vi "Phasor Explorer.vi"() -> ()   [LabVIEW 2019]
uses:
  Decay & Gates Options.ctl
  SEPXP Phasor Plot Info.ctl
  Pseudo Phasor Parameters.ctl
  Phasor Explorer Display Parameters.ctl
  Type of Series.ctl
  Phasor Explorer Phasor Parameters.ctl
  Phasor Calculation Type.ctl
  Phasor Type.ctl
  Phasor Explorer Decay Parameters.ctl
  IRF Model.ctl
  Phasor Explorer Gate Parameters.ctl
  Gate Type.ctl
  Phasor Explorer Detector Parameters.ctl
  SEPXP Q [Element].ctl
  SEPXP Q [Event] List.ctl
  PhXP Internal Variables.ctl
  XY Plot Data.ctl
  XY Graph Plot Properties.ctl
  Cursor Info.ctl
  <vilib>/Utility/miscctls.llb/LVPointDoubleTypeDef.ctl
  SEPXP Globals.vi
  Notebook Main VI Name.vi
  User-defined Gate.vi
  Plot Editor.lvlib
  Notebook.lvlib
  XY Graph Add-Ons.lvlib
  Rich Text Box.lvlib
  Variant to Data.lvlib
panel:
  in  "Abort":bool
  in  "Message":string
  in  "Animated Busy Icon":bool=TRUE
  in  "Display Tabs":T1(tab)
  in  "Show UC Ticks":bool
  out "original tau_m":dbl[unit] format="%#_5g"
  out "original  tau_ph":dbl[unit] format="%#_5g"
  out "Phasor Graph TipStrip":string
  out "current tau_m":dbl[unit] format="%#_5g"
  out "current tau_ph":dbl[unit] format="%#_5g"
  out "tau_i":dbl[unit] format="%#_5g"
  out "Phasor Graph":cluster{"X Array":dbl[], "Y Array":dbl[]}[](graph)
  out "f(tau) Graph TipStrip":string
  out "Numerical Solution":T2 {"Solution 2" format="%#_5g"; "Solution 1" format="%#_5g"}
  out "Analytical Solutions":T2 caption="Analytical Solution" {"Solution 2" format="%#_5g"; "Solution 1" format="%#_5g"}
  in  "Use Cursor":bool caption="Use Pseudo Phasor Graph Cursor"
  in  "Linear Coefficients":cluster{"u":dbl, "v":dbl} {"v" format="%#_5g"; "u" format="%#_5g"}
  out "f(tau) Graph":cluster{"X Array":dbl[], "Y Array":dbl[]}[](graph)
  out "a(b) Graph TipStrip":string
  out "Max Tau":dbl[unit] format="%#_5g"
  out "Min Tau":dbl[unit] format="%#_5g"
  out "a(b) Graph":cluster{"X Array":dbl[], "Y Array":dbl[]}[](graph)=[{"X Array"=[0.0, 0.01, 0.02, 0.03, 0.04, 0.05, 0.060000000000000005, 0.07, 0.08, 0.09, 0.09999999999999999, 0.10999999999999999, 0.11999999999999998, 0.12999999999999998, 0.13999999999999999, 0.15, 0.16, 0.17, 0.18000000000000002, 0.19000000000000003, 0.20000000000000004, 0.21000000000000005, 0.22000000000000006, 0.23000000000000007, 0.24000000000000007, 0.25000000000000006, 0.26000000000000006, 0.2700000000000001, 0.2800000000000001, 0.2900000000000001, 0.3000000000000001, 0.3100000000000001, 0.3200000000000001, 0.3300000000000001, 0.34000000000000014, 0.35000000000000014, 0.36000000000000015, 0.37000000000000016, 0.38000000000000017, 0.3900000000000002, 0.4000000000000002, 0.4100000000000002, 0.4200000000000002, 0.4300000000000002, 0.4400000000000002, 0.45000000000000023, 0.46000000000000024, 0.47000000000000025, 0.48000000000000026, 0.49000000000000027, 0.5000000000000002, 0.5100000000000002, 0.5200000000000002, 0.5300000000000002, 0.5400000000000003, 0.5500000000000003, 0.5600000000000003, 0.5700000000000003, 0.5800000000000003, 0.5900000000000003, 0.6000000000000003, 0.6100000000000003, 0.6200000000000003, 0.6300000000000003, 0.6400000000000003, 0.6500000000000004, 0.6600000000000004, 0.6700000000000004, 0.6800000000000004, 0.6900000000000004, 0.7000000000000004, 0.7100000000000004, 0.7200000000000004, 0.7300000000000004, 0.7400000000000004, 0.7500000000000004, 0.7600000000000005, 0.7700000000000005, 0.7800000000000005, 0.7900000000000005, 0.8000000000000005, 0.8100000000000005, 0.8200000000000005, 0.8300000000000005, 0.8400000000000005, 0.8500000000000005, 0.8600000000000005, 0.8700000000000006, 0.8800000000000006, 0.8900000000000006, 0.9000000000000006, 0.9100000000000006, 0.9200000000000006, 0.9300000000000006, 0.9400000000000006, 0.9500000000000006, 0.9600000000000006, 0.9700000000000006, 0.9800000000000006, 0.9900000000000007, 1.0000000000000007], "Y Array"=[0.0, 0.01, 0.02, 0.03, 0.04, 0.05, 0.060000000000000005, 0.07, 0.08, 0.09, 0.09999999999999999, 0.10999999999999999, 0.11999999999999998, 0.12999999999999998, 0.13999999999999999, 0.15, 0.16, 0.17, 0.18000000000000002, 0.19000000000000003, 0.20000000000000004, 0.21000000000000005, 0.22000000000000006, 0.23000000000000007, 0.24000000000000007, 0.25000000000000006, 0.26000000000000006, 0.2700000000000001, 0.2800000000000001, 0.2900000000000001, 0.3000000000000001, 0.3100000000000001, 0.3200000000000001, 0.3300000000000001, 0.34000000000000014, 0.35000000000000014, 0.36000000000000015, 0.37000000000000016, 0.38000000000000017, 0.3900000000000002, 0.4000000000000002, 0.4100000000000002, 0.4200000000000002, 0.4300000000000002, 0.4400000000000002, 0.45000000000000023, 0.46000000000000024, 0.47000000000000025, 0.48000000000000026, 0.49000000000000027, 0.5000000000000002, 0.5100000000000002, 0.5200000000000002, 0.5300000000000002, 0.5400000000000003, 0.5500000000000003, 0.5600000000000003, 0.5700000000000003, 0.5800000000000003, 0.5900000000000003, 0.6000000000000003, 0.6100000000000003, 0.6200000000000003, 0.6300000000000003, 0.6400000000000003, 0.6500000000000004, 0.6600000000000004, 0.6700000000000004, 0.6800000000000004, 0.6900000000000004, 0.7000000000000004, 0.7100000000000004, 0.7200000000000004, 0.7300000000000004, 0.7400000000000004, 0.7500000000000004, 0.7600000000000005, 0.7700000000000005, 0.7800000000000005, 0.7900000000000005, 0.8000000000000005, 0.8100000000000005, 0.8200000000000005, 0.8300000000000005, 0.8400000000000005, 0.8500000000000005, 0.8600000000000005, 0.8700000000000006, 0.8800000000000006, 0.8900000000000006, 0.9000000000000006, 0.9100000000000006, 0.9200000000000006, 0.9300000000000006, 0.9400000000000006, 0.9500000000000006, 0.9600000000000006, 0.9700000000000006, 0.9800000000000006, 0.9900000000000007, 1.0000000000000007]}]
  in  "Compute Delta Tau":bool
  out "Pseudo-Phase Lifetime Graph TipStrip":string
  out "Pseudo-Phase Lifetime Graph":cluster{"X Array":dbl[], "Y Array":dbl[]}[](graph)=[{"X Array"=[0.0, 1.0, 2.0, 3.0, 4.0, 5.0, 6.0, 7.0, 8.0, 9.0, 10.0, 11.0, 12.0, 13.0, 14.0, 15.0, 16.0, 17.0, 18.0, 19.0, 20.0, 21.0, 22.0, 23.0, 24.0, 25.0, 26.0, 27.0, 28.0, 29.0, 30.0, 31.0, 32.0, 33.0, 34.0, 35.0, 36.0, 37.0, 38.0, 39.0, 40.0, 41.0, 42.0, 43.0, 44.0, 45.0, 46.0, 47.0, 48.0, 49.0, 50.0, 51.0, 52.0, 53.0, 54.0, 55.0, 56.0, 57.0, 58.0, 59.0, 60.0, 61.0, 62.0, 63.0, 64.0, 65.0, 66.0, 67.0, 68.0, 69.0, 70.0, 71.0, 72.0, 73.0, 74.0, 75.0, 76.0, 77.0, 78.0, 79.0, 80.0, 81.0, 82.0, 83.0, 84.0, 85.0, 86.0, 87.0, 88.0, 89.0, 90.0, 91.0, 92.0, 93.0, 94.0, 95.0, 96.0, 97.0, 98.0, 99.0, 100.0], "Y Array"=[0.0, 1.0, 2.0, 3.0, 4.0, 5.0, 6.0, 7.0, 8.0, 9.0, 10.0, 11.0, 12.0, 13.0, 14.0, 15.0, 16.0, 17.0, 18.0, 19.0, 20.0, 21.0, 22.0, 23.0, 24.0, 25.0, 26.0, 27.0, 28.0, 29.0, 30.0, 31.0, 32.0, 33.0, 34.0, 35.0, 36.0, 37.0, 38.0, 39.0, 40.0, 41.0, 42.0, 43.0, 44.0, 45.0, 46.0, 47.0, 48.0, 49.0, 50.0, 51.0, 52.0, 53.0, 54.0, 55.0, 56.0, 57.0, 58.0, 59.0, 60.0, 61.0, 62.0, 63.0, 64.0, 65.0, 66.0, 67.0, 68.0, 69.0, 70.0, 71.0, 72.0, 73.0, 74.0, 75.0, 76.0, 77.0, 78.0, 79.0, 80.0, 81.0, 82.0, 83.0, 84.0, 85.0, 86.0, 87.0, 88.0, 89.0, 90.0, 91.0, 92.0, 93.0, 94.0, 95.0, 96.0, 97.0, 98.0, 99.0, 100.0]}]
  out "Decay & Gates Graph TipStrip":string
  in  "Decay & Gates Options":T3
  out "Decay & Gates Graph":cluster{"X Array":dbl[], "Y Array":dbl[]}[](graph)
  in  "Version":enum32{"Version 1", "Version 2"}(radio)=enum."Version 2"
  out "Sum of Gates Graph TipStrip":string
  out "Sum of Gates Graph":cluster{"X Array":dbl[], "Y Array":dbl[]}[](graph)
  out "Phasor Graph Plots Metadata":T4[](array[typedef]) {"Phasor Explorer Parameters"."Detector Parameters"."Frames/Image" min=1; "Phasor Explorer Parameters"."Detector Parameters"."Multiplicity" min=0; "Phasor Explorer Parameters"."Detector Parameters"."Bits/Frame" min=1; "Phasor Explorer Parameters"."Detector Parameters"."Gates/Frame" min=1; "Phasor Explorer Parameters"."Gate Parameters"."# Steps" min=0.0; "Phasor Explorer Parameters"."Gate Parameters"."Tolerance" min=0.0; "Phasor Explorer Parameters"."Gate Parameters"."Top Slope" min=0.0; "Phasor Explorer Parameters"."Gate Parameters"."Edge Width" min=0.0; "Phasor Explorer Parameters"."Gate Parameters"."Gate Step" min=0.0; "Phasor Explorer Parameters"."Gate Parameters"."# Gates" min=0.0 step=1.0; "Phasor Explorer Parameters"."Gate Parameters"."Gate Width" min=0.0; "Phasor Explorer Parameters"."Decay & IRF Parameters"."Lifetime" min=0.0; "Phasor Explorer Parameters"."Decay & IRF Parameters"."Laser Period" min=0.0; "Phasor Explorer Parameters"."Phasor Parameters"."Square Gate Width" min=0.0; "Phasor Explorer Parameters"."Phasor Parameters"."# Gates" min=0.0; "Phasor Explorer Parameters"."Phasor Parameters"."Calibration Lifetime" min=0.0; "Phasor Explorer Parameters"."Phasor Parameters"."Harmonic frequency" min=0.0; "Phasor Explorer Parameters"."Display Parameters"."Min tau" min=0.0; "Phasor Explorer Parameters"."Display Parameters"."Max tau" min=0.0; "Phasor Explorer Parameters"."Display Parameters"."# Points" min=1 step=1}
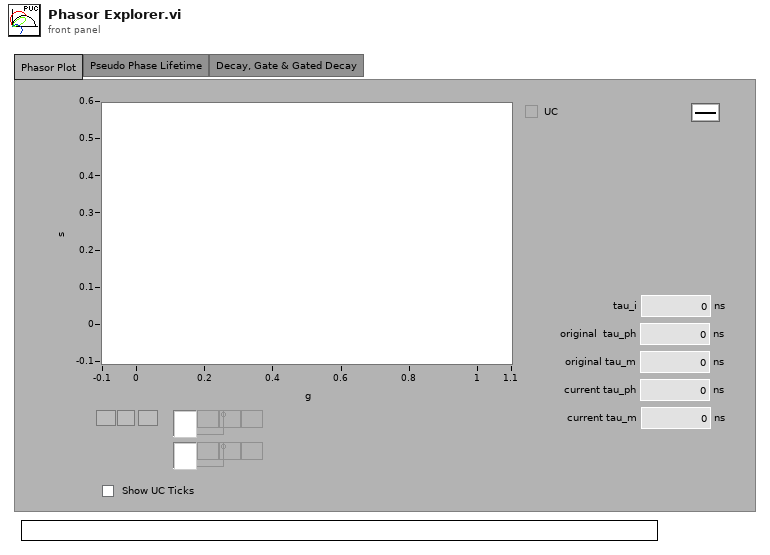
[diagram p1: front panel]
types:
  T1 = enum32{"Phasor Plot", "UC Intersections", "Alpha vs Beta", "Pseudo Phase Lifetime", "Decay, Gate & Gated Decay", "Sum of Gates", "Debug"}
  T2 = cluster{"Solution 1":dbl[unit], "Solution 2":dbl[unit]}
  T3 = typedef "Decay & Gates Options.ctl" = cluster{"Decay":bool, "Gate":bool, "Gated Decay":bool}
  T4 = typedef "SEPXP Phasor Plot Info.ctl" = cluster{"Lifetime/Fraction Array":dbl[], "Phasor Explorer Parameters":T5, "Phase Lifetimes":dbl[], "Modulus Lifetimes":dbl[]}
  T5 = typedef "Pseudo Phasor Parameters.ctl" = cluster{"Display Parameters":T6, "Phasor Parameters":T8, "Decay & IRF Parameters":T11, "Gate Parameters":T13, "Detector Parameters":T15}
  T6 = typedef "Phasor Explorer Display Parameters.ctl" = cluster{"# Points":i32, "Ramp Type":enum16{"Linear", "Logarithmic"}, "Type of Series":T7, "Min tau":dbl[unit], "Max tau":dbl[unit], "Include 0":bool, "Include Infinity":bool}
  T7 = typedef "Type of Series.ctl" = enum16{"1-Exp Decays", "Linear Combination of 1-Exp"}
  T8 = typedef "Phasor Explorer Phasor Parameters.ctl" = cluster{"Harmonic frequency":dbl[unit], "Use f* = 1/D Frequency":bool, "Calibrated Phasor":bool, "Calibration Lifetime":dbl[unit], "Phasor Calculation":T9, "SEPL Type":T10, "# Gates":dbl, "Square Gate Width":dbl[unit], "Show Ticks":bool}
  T9 = typedef "Phasor Calculation Type.ctl" = enum16{"Direct Sum", "Analytical Formula"}
  T10 = typedef "Phasor Type.ctl" = enum16{"UC", "L_N", "L_N[W]"}
  T11 = typedef "Phasor Explorer Decay Parameters.ctl" = cluster{"Lifetime":dbl[unit], "IRF Offset":dbl[unit], "Laser Period":dbl[unit], "Normalized Decays":bool, "IRF Model":T12, "IRF Parameter 1":dbl[unit]}
  T12 = typedef "IRF Model.ctl" = enum16{"Dirac", "Exponential"}
  T13 = typedef "Phasor Explorer Gate Parameters.ctl" = cluster{"First Gate Start":dbl[unit], "Use Gate Center":bool, "Gate Width":dbl[unit], "Gate Step":dbl[unit], "# Gates":dbl, "Gate Type":T14, "Edge Width":dbl[unit], "Top Slope":dbl[unit], "Reversed Sawtooth?":bool, "Analytical Computation":bool, "Tolerance":dbl, "Integration":enum32{"Item 0", "Item 1"}, "# Steps":dbl, "Type of User-defined Function":enum32{"Gate", "IRF"}}
  T14 = typedef "Gate Type.ctl" = enum16{"Square", "Finite Edge Square", "Finite Edge, Tilted Top Square", "Triangle", "Sawtooth", "User-defined"}
  T15 = typedef "Phasor Explorer Detector Parameters.ctl" = cluster{"Frames/Image":i32, "Gates/Frame":i32, "Bits/Frame":i32, "Multiplicity":i32, "Incident Signal":dbl}
  T16 = enum32{"Phasor Plot", "UC Intersections", "Alpha vs Beta", "Pseudo Phase Lifetime", "Decay, Gate & Gated Decay", "Sum of Gates", "Debug"}[]
  T17 = typedef "PhXP Internal Variables.ctl" = cluster{"User-Defined Gate":T18, "User-defined Gate Plot Style":T19}
  T18 = typedef "XY Plot Data.ctl" = cluster{"X Array":dbl[], "Y Array":dbl[]}
  T19 = typedef "XY Graph Plot Properties.ctl" = cluster{"Plot Index":i32, "Plot.Bar Plot Style":u8, "Plot.DigitalLineStyle":u8, "Plot.TransitionLocation":u8, "Plot.Transition Type":u8, "Plot.Fill To":i16, "Plot.Fill/Pt. Color":u32, "Plot.Label Format":u8, "Plot.Line Style":u8, "Plot.Line Width":u8, "Plot.Plot Color":u32, "Plot.Plot Interpolation":u8, "Plot.Plot Name":string, "Plot.Point Style":u8, "Plot.Visible?":bool, "Plot.XScaleIdx":u32, "Plot.YScaleIdx":u32, "Plot.Anti-aliased":bool}
  T20 = typedef "SEPXP Q [Element].ctl" = cluster{"SEPXP Q Event":T21, "Data":variant}
  T21 = typedef "SEPXP Q [Event] List.ctl" = enum16{"Idle", "Initialization", "Show-Hide UC Ticks", "Edit User-defined Gate", "Update Phasor Graph", "Update Sum of Gates Graph", "Update Parameters", "Compute Decay &/or Gates", "Find Pseudo UC Intersections", "Compute alpha(beta) Plot", "Compute Pseudo-Phase Lifetime Plot", "Export Parameters to Clipboard", "Update Phase & Modulus Lifetime", "XY Graph Special Event", "Update Graph Plots Info", "Fit to Circle", "Quit"}
  T22 = typedef "SEPXP Tipstrip Event Registration Refnums.ctl" = cluster{"Phasor Graph Event Registration Refnum":refnum<event-registration>, "Sum of Gates Graph Event Registration Refnum":refnum<event-registration>, "f(tau) Graph Event Registration Refnum":refnum<event-registration>, "a(b) Graph Event Registration Refnum":refnum<event-registration>, "Pseudo-Phase Lifetime Graph Event Registration Refnum":refnum<event-registration>, "Decay & Gate Graph Event Registration Refnum":refnum<event-registration>}
  T23 = enum32{"Phasor Plot", "UC Intersections", "Alpha vs Beta", "Pseudo Phase Lifetime", "Decay, Gate & Gated Decay", "Sum of Gates"}
  T24 = typedef "Cursor Info.ctl" = cluster{"CtlRef":refnum<vi>, "CursIdx":i32, "CursRef":refnum<vi>, "PlotIdx":i32, "PointIdx":i32, "CursLoc":cluster{"X":dbl, "Y":dbl}}
  T25 = typedef "XY Graph Event.ctl" = cluster{"ItemTag":string, "CtlRef":refnum<vi>, "Coords":T26}
  T26 = typedef "LVPoint32TypeDef.ctl" = cluster{"Horizontal":i32, "Vertical":i32}
  T27 = typedef "LVPointDoubleTypeDef.ctl" = cluster{"X":dbl, "Y":dbl}
  T28 = cluster{"XY Graph Ref":refnum<vi>, "Mouse Coordinates":T27, "Plot Index":i32}
  T29 = typedef "Rich Text Box.lvlib/Text Formatting.ctl" = cluster{"Font":string, "Text Color":T30, "Text Background Color":T30, "Text Style":enum16{"Regular", "Bold", "Italic", "Underline", "Strikeout"}, "Font Size (Points)":dbl, "Text Alignment":i32}
  T30 = typedef "Rich Text Box.lvlib/Text Colors.ctl" = enum16{"Unchanged", "Black", "Blue", "Gray", "Green", "Red", "White"}
  T31 = cluster{"ItemTag":string, "CtlRef":refnum<vi>, "Coords":T26}
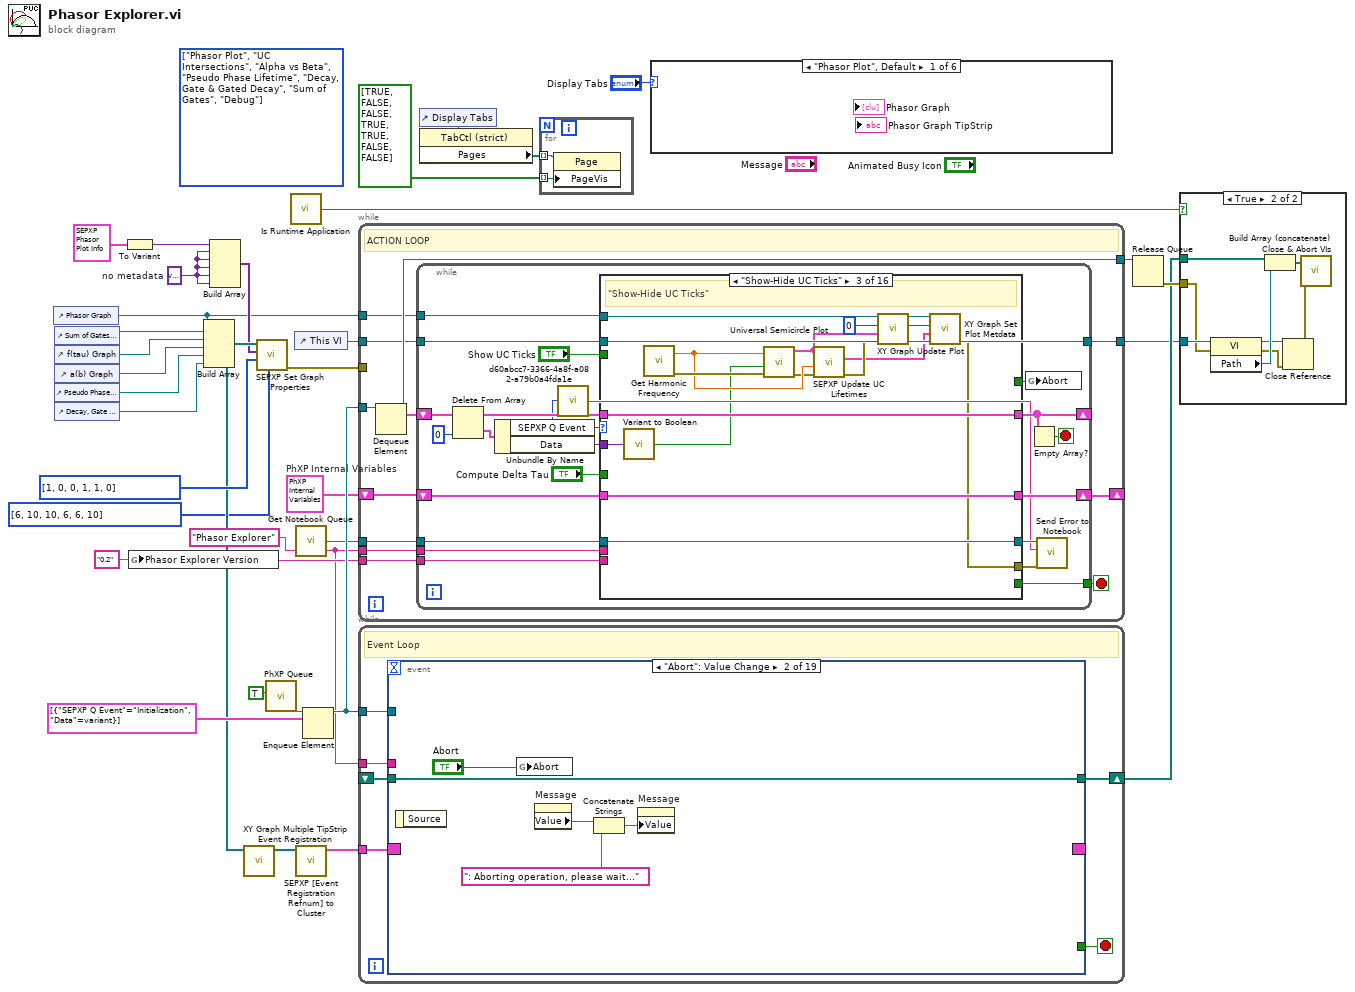
[diagram p0: block diagram]
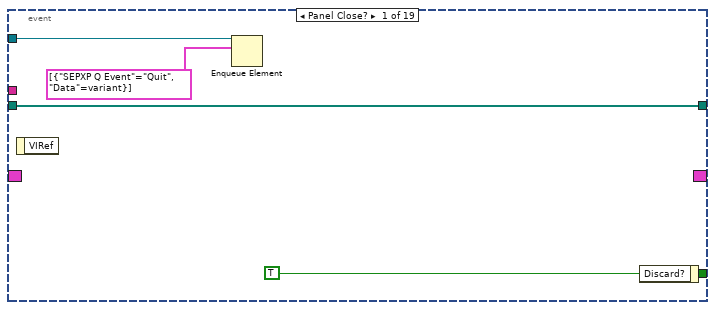
[diagram p3: hidden frame]
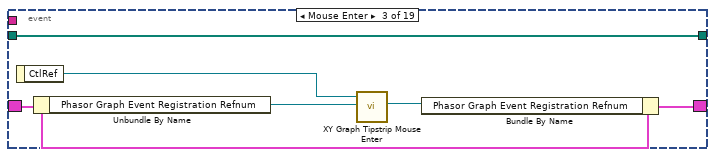
[diagram p4: hidden frame]
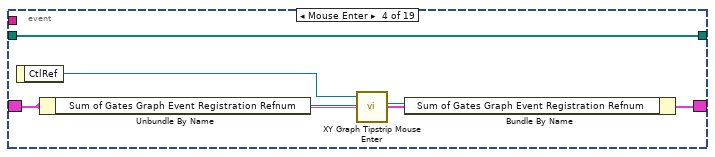
[diagram p5: hidden frame]
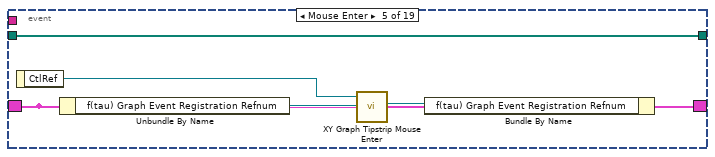
[diagram p6: hidden frame]
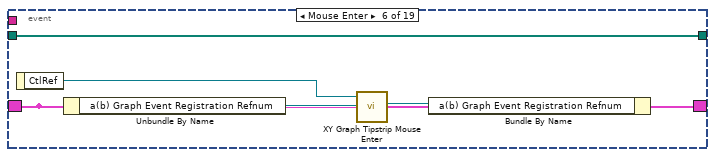
[diagram p7: hidden frame]
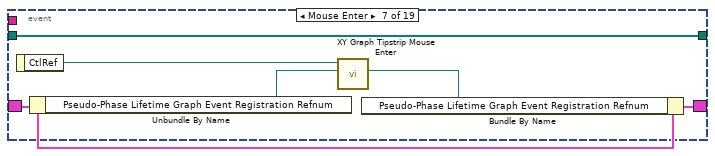
[diagram p8: hidden frame]
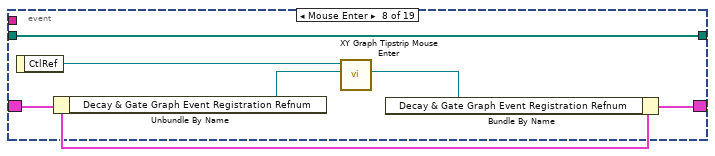
[diagram p9: hidden frame]
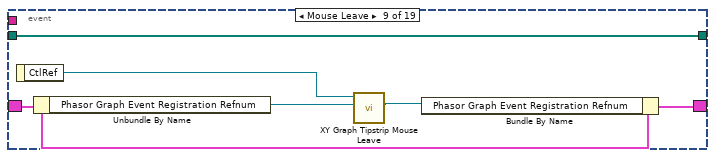
[diagram p10: hidden frame]
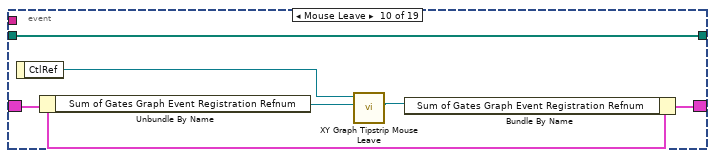
[diagram p11: hidden frame]
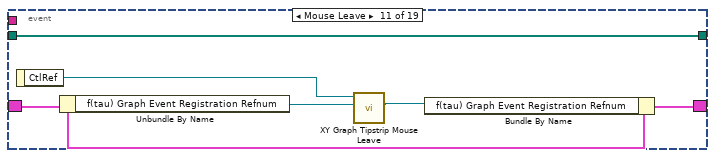
[diagram p12: hidden frame]
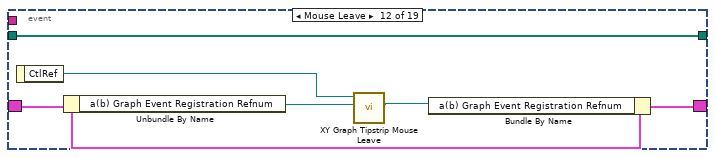
[diagram p13: hidden frame]
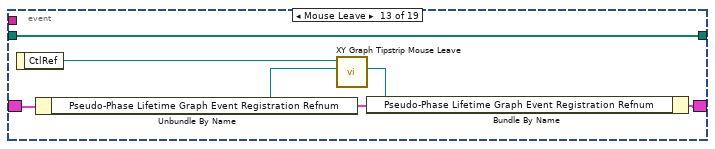
[diagram p14: hidden frame]
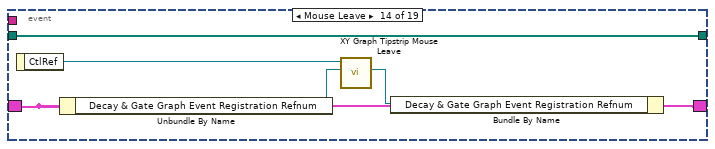
[diagram p15: hidden frame]
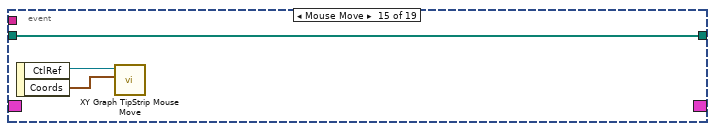
[diagram p16: hidden frame]
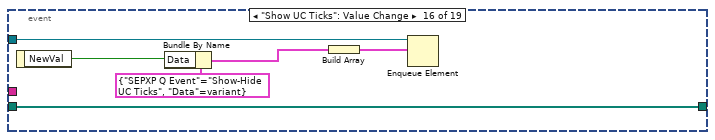
[diagram p17: hidden frame]
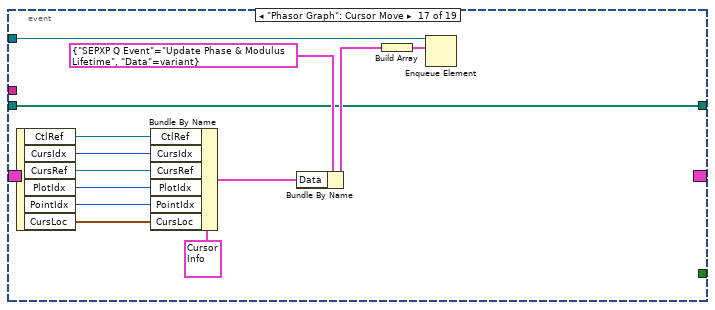
[diagram p18: hidden frame]
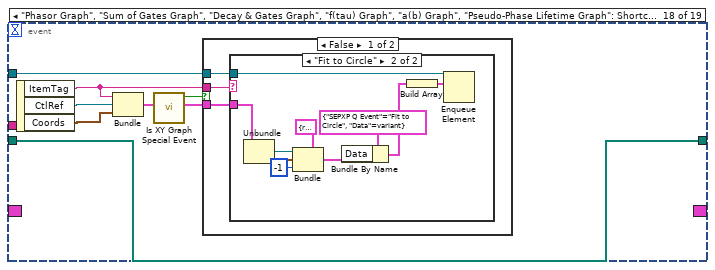
[diagram p19: hidden frame]
diagram:
  (unwired) T16 [enum."Phasor Plot", enum."UC Intersections", enum."Alpha vs Beta", enum."Pseudo Phase Lifetime", enum."Decay, Gate & Gated Decay", enum."Sum of Gates", enum."Debug"] items=["Phasor Plot", "UC Intersections", "Alpha vs Beta", "Pseudo Phase Lifetime", "Decay, Gate & Gated Decay", "Sum of Gates", "Debug"] ("Display Tabs")
  w9 = variant  # no metadata
  w15 = "Phasor Explorer" ("Phasor Explorer Version")
  w28 = "0.2" ("Phasor Explorer Version")
  w31 = T17 {"User-Defined Gate"={"X Array"=[], "Y Array"=[]}, "User-defined Gate Plot Style"={"Plot Index"=0, "Plot.Bar Plot Style"=0, "Plot.DigitalLineStyle"=0, "Plot.TransitionLocation"=0, "Plot.Transition Type"=0, "Plot.Fill To"=-1, "Plot.Fill/Pt. Color"=0, "Plot.Label Format"=0, "Plot.Line Style"=0, "Plot.Line Width"=0, "Plot.Plot Color"=0, "Plot.Plot Interpolation"=4, "Plot.Plot Name"="User-defined Gate", "Plot.Point Style"=0, "Plot.Visible?"=TRUE, "Plot.XScaleIdx"=0, "Plot.YScaleIdx"=0, "Plot.Anti-aliased"=TRUE}}  # PhXP Internal Variables
  n1 = control-ref of="Phasor Graph"() -> (w8:refnum<vi>)
  n2 = control-ref of="Sum of Gates Graph"() -> (w26:refnum<vi>)
  n3 = control-ref of="f(tau) Graph"() -> (w25:refnum<vi>)
  n4 = control-ref of="a(b) Graph"() -> (w24:refnum<vi>)
  n5 = control-ref of="Pseudo Phase Lifetime Graph"() -> (w23:refnum<vi>)
  n6 = control-ref of="Decay, Gate & Gated Decay Graph"() -> (w22:refnum<vi>)
  n7 = To Variant(anything=T4 {"Lifetime/Fraction Array"=[], "Phasor Explorer Parameters"={"Display Parameters"={"# Points"=0, "Ramp Type"=enum."Linear", "Type of Series"=enum."1-Exp Decays", "Min tau"=0.0, "Max tau"=0.0, "Include 0"=FALSE, "Include Infinity"=FALSE}, "Phasor Parameters"={"Harmonic frequency"=0.0, "Use f* = 1/D Frequency"=FALSE, "Calibrated Phasor"=FALSE, "Calibration Lifetime"=1e-09, "Phasor Calculation"=enum."Direct Sum", "SEPL Type"=enum."UC", "# Gates"=1.0, "Square Gate Width"=1e-09, "Show Ticks"=FALSE}, "Decay & IRF Parameters"={"Lifetime"=0.0, "IRF Offset"=0.0, "Laser Period"=0.0, "Normalized Decays"=FALSE, "IRF Model"=enum."Dirac", "IRF Parameter 1"=0.0}, "Gate Parameters"={"First Gate Start"=0.0, "Use Gate Center"=FALSE, "Gate Width"=0.0, "Gate Step"=0.0, "# Gates"=0.0, "Gate Type"=enum."Square", "Edge Width"=0.0, "Top Slope"=0.0, "Reversed Sawtooth?"=FALSE, "Analytical Computation"=FALSE, "Tolerance"=1.0, "Integration"=enum."Item 0", "# Steps"=1.0, "Type of User-defined Function"=enum."Gate"}, "Detector Parameters"={"Frames/Image"=0, "Gates/Frame"=0, "Bits/Frame"=0, "Multiplicity"=0, "Incident Signal"=0.0}}, "Phase Lifetimes"=[], "Modulus Lifetimes"=[]} ("Phasor Graph Plot Info")) -> (Variant=w11:variant)
  n8 = global write "SEPXP Globals.vi" "Phasor Explorer Version"(w28) -> ()
  n9 = Build Array(w8, w26, w25, w24, w23, w22) -> (w19:refnum<vi>[])
  n10 = Build Array(w11, w9, w9, w9, w9, w9) -> (w10:variant[])
  n11 = call "XY Graph Multiple TipStrip Event Registration.vi"("XY Graph Refnums"=w19) -> ("Tipstrips Event Registrations"=w18:refnum<event-registration>[])  [unwired: 9 in, 1 out]
  n12 = call "SEPXP Set Graph Properties.vi"("Max Legend Size (8)"=i32[] [6, 10, 10, 6, 6, 10], "# Preserved PLots"=i32[] [1, 0, 0, 1, 1, 0], "Metadata Type"=w10, "XY Graph Ref Array"=w19) -> ("Error Out"=w21:errorcluster)  [unwired: 7 in]
  n13 = call "PhXP Queue.vi"("create if not found? (F)"=TRUE) -> ("PhXP Queue"=w14:refnum<queue>)  [unwired: 10 in]
  n14 = call "Is Runtime Application.vi"() -> ("Runtime ?"=w2:bool)  [unwired: 8 in, 1 out]
  n15 = control-ref of="This VI"() -> (w7:refnum<vi>)
  n16 = call "Get Notebook Queue.vi"() -> ("Notebook Queue"=w29:refnum<queue>)  [unwired: 9 in]
  n17 = call "SEPXP [Event Registration Refnum] to Cluster.vi"("Tipstrips Event Registrations"=w18) -> ("Tipstrip RE refnums"=w17:T22)  [unwired: 10 in]
  n18 = Enqueue Element(queue=w14, element=T20[] [{"SEPXP Q Event"=enum."Initialization", "Data"=variant}] ("PSEXP Q Element")) -> (queue out=w32:refnum<queue>)  [unwired: 2 in, 2 out]
  n19 = while {
    tunnel: w32 -> [w46]
    tunnel: [w44] -> w33
    tunnel: w7 -> [w42]
    shift-right: [w40] -> _
    shift-left: w31 -> [w41]
    tunnel: w29 -> [w39]
    tunnel: w28 -> [w38]
    tunnel: w15 -> [w37]
    tunnel: w21 -> [_]
    tunnel: w8 -> [w36]
    tunnel: [w35] -> w1
    stop <- w43 stop-if-true
    # "ACTION LOOP"
    n20 = Dequeue Element(queue=w46) -> (queue out=w44:refnum<queue>, element=w45:T20[])  [unwired: 2 in, 2 out]
    n21 = while {
      shift-right: [w64] -> _
      shift-left: w45 -> [w66]
      tunnel: [w62] -> w43
      tunnel: w42 -> [w47]
      shift-right: [w60] -> w40
      shift-left: w41 -> [w61]
      tunnel: w39 -> [w58]
      tunnel: w38 -> [w57]
      tunnel: w37 -> [w56]
      tunnel: w36 -> [w50]
      tunnel: [w47] -> w35
      stop <- w63 stop-if-true
      n22 = Delete From Array(array=w66, index=0) -> (deleted portion=w67:T20, array with subset deleted=w65:T20[])  [unwired: 1 in]
      n23 = Unbundle By Name(w67) -> ("SEPXP Q Event"=w52:T21, "Data"=w59:variant)
      n24 = call "d60abcc7-3366-4a8f-a082-a79b0a4fda1e.vi"("Enum"=w52) -> ("String"=w51:string)
      n25 = case shown="\"Show-Hide UC Ticks\"" w52 {
        tunnel: w65 -> [w71 w93 w121 w131 w144 w152 w164 w176 w185 w191 w201 w223 w232 w239 w250 _]
        tunnel: [w71 w93 w121 w131 w144 w152 w164 w176 w185 w191 w201 w223 w232 w239 w250 T20[] []] -> w64
        tunnel: [_ _ _ _ _ _ _ _ _ _ _ _ _ _ _ w252] -> w62
        tunnel: w47 -> [_ _ _ _ w141 w148 _ w167 w180 _ w195 w219 _ _ _ _]
        tunnel: w61 -> [w70 w77 w119 w128 w136 w149 w158 w173 w182 w188 w196 w220 w231 w238 w249 w258]
        tunnel: [w70 w77 w119 w129 w136 w149 w158 w173 w182 w188 w196 w220 w231 w238 w249 w258] -> w60
        tunnel: w59 -> [_ _ w108 _ _ _ w163 _ _ _ _ _ w228 _ w248 _]
        tunnel: w58 -> [w69 w84 w120 w122 w137 w145 w156 w165 w177 w186 w192 w202 w224 w237 w245 w254]
        tunnel: w57 -> [_ w92 _ _ _ _ _ _ _ _ _ _ _ _ _ w256]
        tunnel: w56 -> [_ w91 _ _ _ _ _ _ _ _ _ _ _ _ _ w257]
        tunnel: "Compute Delta Tau" -> [_ _ _ _ _ _ _ _ w179 _ _ _ _ _ _ _]
        tunnel: [_ w86 w112 w123 w138 w146 w157 w166 w178 w187 w193 w203 w225 _ w243 w251] -> w54
        tunnel: [w69 w84 w120 w122 w137 w145 w156 w165 w177 w186 w192 w202 w224 w237 w245 w254] -> w53
        tunnel: w50 -> [_ w82 w114 _ _ _ _ _ _ _ _ _ _ w236 _ _]
        tunnel: [_ _ _ _ FALSE ("Abort") _ _ _ _ _ _ _ _ _ _ _] -> w49
        tunnel: "Show UC Ticks" -> [_ w72 _ _ _ _ _ _ _ _ _ _ _ _ _ _]
        frame "Idle", Default {
          # "\"Idle\", Default"
        }
        frame "Initialization" {
          # "\"Initialization\""
          n26 = call "Send Start-Stop Message.vi"("Start(T)/Stop(F)"=TRUE, "Version number"=w92, "Software Name"=w91, "Notebook Queue"=w84) -> ("Error Out"=w85:errorcluster)  [unwired: 7 in]
          n27 = call "Save-Load PhXP Settings.vi"("Load(F)/Save (T)"=FALSE) -> ("Error Out"=w89:errorcluster)  [unwired: 9 in, 1 out]
          n28 = call "9d87ee79-5232-47ce-8c93-ac6730099a75.vi"("# Steps (1)"=100) -> ("Ramp"=w101:dbl[])  [unwired: 9 in, 1 out]
          n29 = call "79f5c63b-0c71-4b9b-95d4-cbcc2b15c9cb.vi"("# Steps (1)"=100, "End (1)"=100.0) -> ("Ramp"=w106:dbl[])  [unwired: 8 in, 1 out]
          n30 = call "Get Harmonic Frequency.vi"("Error In"=w89) -> ("Error Out"=w75:errorcluster, "Harmonic frequency"=w76:dbl[unit])  [unwired: 2 in, 1 out]
          n31 = Bundle("Ramp"=w101, "Ramp"=w101) -> (w103:cluster{"Ramp":dbl[], "Ramp":dbl[]})  [unwired: 1 in]
          n32 = Bundle("Ramp"=w106, "Ramp"=w106) -> (w104:cluster{"Ramp":dbl[], "Ramp":dbl[]})  [unwired: 1 in]
          n33 = call "Universal Semicircle Plot.vi"("Error In"=w75, "Show Ticks"=w72, "Harmonic frequency"=w76) -> ("Error Out"=w74:errorcluster, "Universal Semi-circle"=w80:cluster{"X Array":dbl[], "Y Array":dbl[]})  [unwired: 6 in, 1 out]
          n34 = Build Array(w103) -> (w102:cluster{"Ramp":dbl[], "Ramp":dbl[]}[])
          n35 = Build Array(w104) -> (w105:cluster{"Ramp":dbl[], "Ramp":dbl[]}[])
          n36 = call "SEPXP Update UC Lifetimes.vi"("Error In"=w74, "Harmonic Frequency"=w76, "Universal Semi-circle"=w80) -> ("Error Out"=w73:errorcluster, "PhXP UC Plot Info out"=w81:T4)  [unwired: 7 in]
          n37 = property on="a(b) Graph" class="XYGraph (strict)"("Value"=w102, "Active Plot"=u32 0, "Plot.Plot Name"="alpha = beta") -> ()  [unwired: 2 in, 2 out]
          n38 = property on="Pseudo-Phase Lifetime Graph" class="XYGraph (strict)"("Value"=w105, "Active Plot"=u32 0, "Plot.Plot Name"="tau = P-tau_ph") -> ()  [unwired: 2 in, 2 out]
          n39 = call "XY Graph Add Single Plot with Name.vi"("XYGraph Ref in"=w82, "Keep Existing Plots (T)"=FALSE, "Plot"=w80, "Plot Metadata"=w81, "Plot Name (\"Plot\")"="UC" ("Plot.Plot Name"), "error in (no error)"=w73) -> ("error out"=w78:errorcluster)  [unwired: 6 in, 3 out]
          n40 = Merge Errors(w78, w85) -> (w86:errorcluster)
          n41 = local write "Display Tabs"(T23."Phasor Plot" ("Display Tabs")) -> ()
        }
        frame "Show-Hide UC Ticks" {
          w111 = 0 ("Plot Idx")
          # "\"Show-Hide UC Ticks\""
          n42 = call "Variant to Boolean.vi"("Variant"=w108) -> ("Value"=w107:bool)  [unwired: 8 in]
          n43 = call "Get Harmonic Frequency.vi"() -> ("Error Out"=w118:errorcluster, "Harmonic frequency"=w117:dbl[unit])  [unwired: 3 in, 1 out]
          n44 = call "Universal Semicircle Plot.vi"("Error In"=w118, "Show Ticks"=w107, "Harmonic frequency"=w117) -> ("Error Out"=w116:errorcluster, "Universal Semi-circle"=w109:cluster{"X Array":dbl[], "Y Array":dbl[]})  [unwired: 6 in, 1 out]
          n45 = call "SEPXP Update UC Lifetimes.vi"("Error In"=w116, "Harmonic Frequency"=w117, "Universal Semi-circle"=w109) -> ("Error Out"=w115:errorcluster, "PhXP UC Plot Info out"=w110:T4)  [unwired: 7 in]
          n46 = call "XY Graph Update Plot.vi"("Error In"=w115, "Plot"=w109, "Plot Idx"=w111, "XY Graph refnum"=w114) -> ("Error Out"=w113:errorcluster)  [unwired: 7 in]
          n47 = call "XY Graph Set Plot Metdata.vi"("error in (no error)"=w113, "Plot Metadata"=w110, "Plot Index (-1: last)"=w111, "XYGraph Ref in"=w114) -> ("error out"=w112:errorcluster)  [unwired: 5 in, 2 out]
        }
        frame "Edit User-defined Gate" {
          # "\"Edit User-defined Gate\""
          n48 = Unbundle By Name(w128) -> ("User-Defined Gate"=w130:T18, "User-defined Gate Plot Style"=w125:T19)
          n49 = call "Plot Editor.vi"("Original Graph Name"="User-Defined Gate/IRF Plot", "Plot Style in"=w125, "Plot in"=w130) -> ("Error Out"=w123:errorcluster, "Plot Style out"=w124:T19, "Plot out"=w127:T18)  [unwired: 6 in]
          n50 = Bundle By Name(cluster=w128, "User-Defined Gate"=w127, "User-defined Gate Plot Style"=w124) -> (w129:T17)
          n51 = global write "User-defined Gate.vi" "User-defined Gate"(w127) -> ()
        }
        frame "Update Phasor Graph" {
          # "\"Update Phasor Graph\""
          n52 = call "Show Animated Busy Icon with Message and Abort Button.vi"("Message"="Computing Phasor Graph...", "Target VI reference"=w141) -> ("Error Out"=w143:errorcluster)  [unwired: 17 in]
          n53 = call "Compute Pseudo UC Wrapper.vi"("error in (no error)"=w143, "VI in"=w141) -> ("error out"=w142:errorcluster, "Notebook String"=w133:string, "Plot Name"=w134:string)  [unwired: 7 in]
          n54 = call "Hide Animated Busy Icon with Message and Abort Button.vi"("Error In"=w142) -> ("Error Out"=w135:errorcluster)  [unwired: 18 in]
          n55 = call "Send PhXP Phasor Plot Info to Notebook.vi"("Graph Type"="Phasor", "error in (no error)"=w135, "Phasor Plot Info String"=w133, "Plot Name"=w134, "Notebook Queue"=w137) -> ("Error Out"=w138:errorcluster)  [unwired: 6 in]
        }
        frame "Update Sum of Gates Graph" {
          # "\"Update Sum of Gates Graph\""
          n56 = call "Show Animated Busy Icon with Message and Abort Button.vi"("Message"="Computing Sum of Gates...", "Target VI reference"=w148) -> ("Error Out"=w151:errorcluster)  [unwired: 17 in]
          n57 = call "Compute Sum of Gates Plot Wrapper.vi"("error in (no error)"=w151, "VI in"=w148) -> ("error out"=w150:errorcluster)  [unwired: 9 in]
          n58 = call "Hide Animated Busy Icon with Message and Abort Button.vi"("Error In"=w150) -> ("Error Out"=w146:errorcluster)  [unwired: 18 in]
        }
        frame "Update Phase & Modulus Lifetime" {
          # "\"Update Phase & Modulus Lifetime\""
          n59 = Variant To Data(Variant=w163) -> (data=w153:T24, error out=w159:errorcluster)  [unwired: 2 in]
          n60 = call "Get tau_i, tau_phi, tau_m at Cursor.vi"("Error In"=w159, "Cursor Info"=w153) -> ("Error Out"=w157:errorcluster, "current tau_m"=→"current tau_m":dbl[unit], "current tau_ph"=→"current tau_ph":dbl[unit], "tau_i"=→"tau_i":dbl[unit], "original tau_ph"=→"original  tau_ph":dbl[unit], "original tau_m"=→"original tau_m":dbl[unit])  [unwired: 4 in]
        }
        frame "Compute Decay &/or Gates" {
          # "\"Compute Decay &/or Gates\""
          n61 = call "Show Animated Busy Icon with Message and Abort Button.vi"("Message"="Computing Decay/Gates...", "Target VI reference"=w167) -> ("Error Out"=w175:errorcluster)  [unwired: 17 in]
          n62 = call "Compute Decay & Time Gates Wrapper.vi"("error in (no error)"=w175, "VI in"=w167) -> ("error out"=w174:errorcluster, "Decay & Gates Plot String"=w171:string, "Added Plot Name(s)"=w168:string)  [unwired: 6 in, 1 out]
          n63 = call "Hide Animated Busy Icon with Message and Abort Button.vi"("Target VI reference"=w167, "Error In"=w174) -> ("Error Out"=w170:errorcluster)  [unwired: 17 in]
          n64 = call "Send PhXP Phasor Plot Info to Notebook.vi"("Graph Type"="Decay & Gates", "error in (no error)"=w170, "Phasor Plot Info String"=w171, "Plot Name"=w168, "Notebook Queue"=w165) -> ("Error Out"=w166:errorcluster)  [unwired: 6 in]
        }
        frame "Compute Pseudo-Phase Lifetime Plot" {
          # "\"Compute Pseudo-Phase Lifetime Plot\""
          n65 = call "Show Animated Busy Icon with Message and Abort Button.vi"("Message"="Computing Phase Lifetime Plot...", "Target VI reference"=w180) -> ("Error Out"=w184:errorcluster)  [unwired: 17 in]
          n66 = call "Compute Pseudo-Phase Lifetime Plot Wrapper.vi"("Compute Delta Tau"=w179, "error in (no error)"=w184, "VI in"=w180) -> ("error out"=w183:errorcluster)  [unwired: 8 in]
          n67 = call "Hide Animated Busy Icon with Message and Abort Button.vi"("Target VI reference"=w180, "Error In"=w183) -> ("Error Out"=w178:errorcluster)  [unwired: 17 in]
        }
        frame "Export Parameters to Clipboard" {
          # "\"Export Parameters to Clipboard\""
          n68 = call "Show Animated Busy Icon.vi"() -> ("Error Out"=w190:errorcluster)  [unwired: 9 in]
          n69 = call "Export Parameters to Clipboard Wrapper.vi"("error in (no error)"=w190) -> ("error out"=w189:errorcluster)  [unwired: 10 in]
          n70 = call "Hide Animated Busy Icon.vi"("Error In"=w189) -> ("Error Out"=w187:errorcluster)  [unwired: 8 in]
        }
        frame "Compute alpha(beta) Plot" {
          # "\"Compute alpha(beta) Plot\""
          n71 = call "Show Animated Busy Icon with Message and Abort Button.vi"("Message"="Computing Alpha(beta) Plot...", "Target VI reference"=w195) -> ("Error Out"=w200:errorcluster)  [unwired: 17 in]
          n72 = call "Compute alpha(beta) Plot Wrapper.vi"("error in (no error)"=w200, "VI in"=w195) -> ("error out"=w199:errorcluster, "Max Tau"=→"Max Tau":dbl[unit], "Min Tau"=→"Min Tau":dbl[unit])  [unwired: 7 in]
          n73 = call "Hide Animated Busy Icon with Message and Abort Button.vi"("Error In"=w199) -> ("Error Out"=w193:errorcluster)  [unwired: 18 in]
        }
        frame "Find Pseudo UC Intersections" {
          # "\"Find Pseudo UC Intersections\""
          n74 = call "Show Animated Busy Icon with Message.vi"("Message"="Computing UC Intersections...", "Target VI reference"=w219) -> ("Error Out"=w222:errorcluster)  [unwired: 9 in]
          n75 = call "Compute f(tau) & Zeros Wrapper.vi"("VI in"=w219, "error in (no error)"=w222) -> ("Numerical Solution 1"=w207:dbl[unit], "Numerical Solution 2"=w206:dbl[unit], "Analytical Solution 1"=w204:dbl[unit], "Analytical Solution 2"=w216:dbl[unit], "error out"=w221:errorcluster)  [unwired: 9 in]
          n76 = Not A Number/Path/Refnum?(number/path/refnum=w216) -> (NaN/Path/Refnum?=w217:bool)
          n77 = Not A Number/Path/Refnum?(number/path/refnum=w204) -> (NaN/Path/Refnum?=w215:bool)
          n78 = Not(x=w217) -> (.not. x?=w213:bool)
          n79 = call "Show Animated Busy Icon with Message and Abort Button.vi"("Error In"=w221) -> ("Error Out"=w203:errorcluster)  [unwired: 18 in]
          n80 = Not(x=w215) -> (.not. x?=w214:bool)
          n81 = Or(x=w214, y=w213) -> (x .or. y?=w212:bool)
          n82 = Not A Number/Path/Refnum?(number/path/refnum=w206) -> (NaN/Path/Refnum?=w211:bool)
          n83 = property on="Analytical Solutions" class="Clust (strict)"("Visible"=w212) -> ()  [unwired: 2 in, 2 out]
          n84 = property on="Solution 2" class="DigNum (strict)"("Value"=w216, "Visible"=w213) -> ()  [unwired: 2 in, 2 out]
          n85 = Not A Number/Path/Refnum?(number/path/refnum=w207) -> (NaN/Path/Refnum?=w210:bool)
          n86 = property on="Solution 1" class="DigNum (strict)"("Value"=w204, "Visible"=w214) -> ()  [unwired: 2 in, 2 out]
          n87 = Not(x=w211) -> (.not. x?=w205:bool)
          n88 = Not(x=w210) -> (.not. x?=w209:bool)
          n89 = Or(x=w209, y=w205) -> (x .or. y?=w208:bool)
          n90 = property on="Solution 1" class="DigNum (strict)"("Value"=w207, "Visible"=w209) -> ()  [unwired: 2 in, 2 out]
          n91 = property on="Solution 2" class="DigNum (strict)"("Value"=w206, "Visible"=w205) -> ()  [unwired: 2 in, 2 out]
          n92 = property on="Numerical Solution" class="Clust (strict)"("Visible"=w208) -> ()  [unwired: 2 in, 2 out]
        }
        frame "XY Graph Special Event" {
          # "\"XY Graph Special Event\""
          n93 = Variant To Data(Variant=w228) -> (data=w229:T25, error out=w230:errorcluster)  [unwired: 2 in]
          n94 = call "XY Graph Special Event Handler Wrapper.vi"("Error In"=w230, "XY Graph Event"=w229) -> ("Error Out"=w226:errorcluster, "Message"=w227:string)  [unwired: 8 in]
          n95 = call "Send Message to Notebook.vi"("Notebook Queue"=w224, "Message"=w227, "Error In"=w226) -> ("Error Out"=w225:errorcluster)  [unwired: 16 in]
        }
        frame "Update Graph Plots Info" {
          # "\"Update Graph Plots Info\""
          n96 = call "XY Graph Get Plots Metadata.vi"("XYGraph Refnum"=w236) -> ("Plots Metadata"=w235:variant[])  [unwired: 7 in, 3 out]
          n97 = Variant To Data(type=T4[] [] ("Array"), Variant=w235) -> (data=→"Phasor Graph Plots Metadata":T4[])  [unwired: 1 in, 1 out]
        }
        frame "Fit to Circle" {
          # "\"Fit to Circle\""
          n98 = Variant To Data(Variant=w248) -> (data=w247:T28, error out=w246:errorcluster)  [unwired: 2 in]
          n99 = call "Fit Plot to Circle.vi"("Full Circle Plot"=FALSE, "Error In"=w246, "Circle Fit Plot Information"=w247) -> ("Error Out"=w244:errorcluster, "Result String"=w242:string)  [unwired: 6 in, 1 out]
          n100 = call "Result Style.vi"() -> ("Default Text Formatting"=w241:T29)
          n101 = call "Send Message to Notebook.vi"("Notebook Queue"=w245, "Message"=w242, "Error In"=w244, "Text Formatting"=w241) -> ("Error Out"=w243:errorcluster)  [unwired: 15 in]
        }
        frame "Quit" {
          w252 = TRUE
          # "\"Quit\""
          n102 = call "Send Start-Stop Message.vi"("Start(T)/Stop(F)"=FALSE, "Version number"=w256, "Software Name"=w257, "Notebook Queue"=w254) -> ("Error Out"=w253:errorcluster)  [unwired: 7 in]
          n103 = call "Save-Load PhXP Settings.vi"("Load(F)/Save (T)"=w252, "Error In"=w253) -> ("Error Out"=w251:errorcluster)  [unwired: 8 in, 1 out]
        }
      }
      n104 = global write "SEPXP Globals.vi" "Abort"(w49) -> ()
      n105 = Empty Array?(array=w64) -> (empty?=w63:bool)
      n106 = call "Send Error to Notebook.vi"("error in (no error)"=w54, "State Machine Case Error Source"=w51, "Notebook Q"=w53) -> ()  [unwired: 9 in]
    }
  }
  n107 = while {
    tunnel: w32 -> [w265]
    tunnel: w17 -> [w263]
    tunnel: w15 -> [w262]
    shift-right: [w261] -> w6
    shift-left: _ -> [w260]
    stop <- w264 stop-if-true
    # "Event Loop"
    n108 = event shown="[1] \"Abort\": Value Change" {
      selector: w263 -> [_ _ w278 w284 w290 w296 w302 w308 w316 w322 w328 w334 w340 w346 _ _ _ _ _]
      dyn-events: [_ _ w276 w282 w288 w294 w300 w306 w315 w321 w327 w333 w339 w345 _ _ _ _ _] -> _
      timeout: _ -> [_ _ _ _ _ _ _ _ _ _ _ _ _ _ _ _ _ _ _]
      tunnel: [w269 _ _ _ _ _ _ _ _ _ _ _ _ _ _ _ _ _ w398] -> w264
      tunnel: w265 -> [w268 _ _ _ _ _ _ _ _ _ _ _ _ _ _ w355 w368 w371 w400]
      tunnel: w262 -> [_ _ _ _ _ _ _ _ _ _ _ _ _ _ _ _ _ _ w397]
      tunnel: [w266 w270 w275 w281 w287 w293 w299 w305 w311 w317 w323 w329 w335 w341 w347 w350 w356 w369 w396] -> w261
      tunnel: w260 -> [w266 w270 w275 w281 w287 w293 w299 w305 w311 w317 w323 w329 w335 w341 w347 w350 w356 w369 w395]
      event Panel Close? {
        w269 = TRUE ("Discard?")
        n109 = event-data() -> ()  [unwired: 1 in, 1 out]
        n110 = Enqueue Element(queue=w268, element=T20[] [{"SEPXP Q Event"=enum."Quit", "Data"=variant}]) -> ()  [unwired: 2 in, 3 out]
        n111 = event-data("Discard?"=w269) -> ()  [unwired: 1 in, 1 out]
      }
      event "Abort": Value Change {
        n112 = event-data() -> ()  [unwired: 1 in, 1 out]
        n113 = global write "SEPXP Globals.vi" "Abort"("Abort") -> ()
        n114 = property on="Message" class="Str"() -> ("Value"=w273:string)  [unwired: 2 in, 2 out]
        n115 = Concatenate Strings(w273, ": Aborting operation, please wait..." ("string")) -> (w271:string)
        n116 = property on="Message" class="Str"("Value"=w271) -> ()  [unwired: 2 in, 2 out]
      }
      event Mouse Enter {
        n117 = event-data() -> ("CtlRef"=w279:refnum<vi>)  [unwired: 1 in]
        n118 = Unbundle By Name(w278) -> ("Phasor Graph Event Registration Refnum"=w280:refnum<event-registration>)
        n119 = call "XY Graph Tipstrip Mouse Enter.vi"("Event Registration Refnum"=w280, "XY Graph Refnum"=w279) -> ("Event Registration Refnum"=w277:refnum<event-registration>)  [unwired: 8 in, 1 out]
        n120 = Bundle By Name(cluster=w278, "Phasor Graph Event Registration Refnum"=w277) -> (w276:T22)
      }
      event Mouse Enter {
        n121 = event-data() -> ("CtlRef"=w285:refnum<vi>)  [unwired: 1 in]
        n122 = Unbundle By Name(w284) -> ("Sum of Gates Graph Event Registration Refnum"=w286:refnum<event-registration>)
        n123 = call "XY Graph Tipstrip Mouse Enter.vi"("Event Registration Refnum"=w286, "XY Graph Refnum"=w285) -> ("Event Registration Refnum"=w283:refnum<event-registration>)  [unwired: 8 in, 1 out]
        n124 = Bundle By Name(cluster=w284, "Sum of Gates Graph Event Registration Refnum"=w283) -> (w282:T22)
      }
      event Mouse Enter {
        n125 = event-data() -> ("CtlRef"=w291:refnum<vi>)  [unwired: 1 in]
        n126 = Unbundle By Name(w290) -> ("f(tau) Graph Event Registration Refnum"=w292:refnum<event-registration>)
        n127 = call "XY Graph Tipstrip Mouse Enter.vi"("Event Registration Refnum"=w292, "XY Graph Refnum"=w291) -> ("Event Registration Refnum"=w289:refnum<event-registration>)  [unwired: 8 in, 1 out]
        n128 = Bundle By Name(cluster=w290, "f(tau) Graph Event Registration Refnum"=w289) -> (w288:T22)
      }
      event Mouse Enter {
        n129 = event-data() -> ("CtlRef"=w297:refnum<vi>)  [unwired: 1 in]
        n130 = Unbundle By Name(w296) -> ("a(b) Graph Event Registration Refnum"=w298:refnum<event-registration>)
        n131 = call "XY Graph Tipstrip Mouse Enter.vi"("Event Registration Refnum"=w298, "XY Graph Refnum"=w297) -> ("Event Registration Refnum"=w295:refnum<event-registration>)  [unwired: 8 in, 1 out]
        n132 = Bundle By Name(cluster=w296, "a(b) Graph Event Registration Refnum"=w295) -> (w294:T22)
      }
      event Mouse Enter {
        n133 = event-data() -> ("CtlRef"=w303:refnum<vi>)  [unwired: 1 in]
        n134 = Unbundle By Name(w302) -> ("Pseudo-Phase Lifetime Graph Event Registration Refnum"=w304:refnum<event-registration>)
        n135 = call "XY Graph Tipstrip Mouse Enter.vi"("Event Registration Refnum"=w304, "XY Graph Refnum"=w303) -> ("Event Registration Refnum"=w301:refnum<event-registration>)  [unwired: 8 in, 1 out]
        n136 = Bundle By Name(cluster=w302, "Pseudo-Phase Lifetime Graph Event Registration Refnum"=w301) -> (w300:T22)
      }
      event Mouse Enter {
        n137 = event-data() -> ("CtlRef"=w309:refnum<vi>)  [unwired: 1 in]
        n138 = Unbundle By Name(w308) -> ("Decay & Gate Graph Event Registration Refnum"=w310:refnum<event-registration>)
        n139 = call "XY Graph Tipstrip Mouse Enter.vi"("Event Registration Refnum"=w310, "XY Graph Refnum"=w309) -> ("Event Registration Refnum"=w307:refnum<event-registration>)  [unwired: 8 in, 1 out]
        n140 = Bundle By Name(cluster=w308, "Decay & Gate Graph Event Registration Refnum"=w307) -> (w306:T22)
      }
      event Mouse Leave {
        n141 = event-data() -> ("CtlRef"=w312:refnum<vi>)  [unwired: 1 in]
        n142 = Unbundle By Name(w316) -> ("Phasor Graph Event Registration Refnum"=w314:refnum<event-registration>)
        n143 = call "XY Graph Tipstrip Mouse Leave.vi"("Event Registration Refnum"=w314, "XY Graph Refnum"=w312) -> ("Event Registration Refnum"=w313:refnum<event-registration>)  [unwired: 8 in, 1 out]
        n144 = Bundle By Name(cluster=w316, "Phasor Graph Event Registration Refnum"=w313) -> (w315:T22)
      }
      event Mouse Leave {
        n145 = event-data() -> ("CtlRef"=w318:refnum<vi>)  [unwired: 1 in]
        n146 = Unbundle By Name(w322) -> ("Sum of Gates Graph Event Registration Refnum"=w320:refnum<event-registration>)
        n147 = call "XY Graph Tipstrip Mouse Leave.vi"("Event Registration Refnum"=w320, "XY Graph Refnum"=w318) -> ("Event Registration Refnum"=w319:refnum<event-registration>)  [unwired: 8 in, 1 out]
        n148 = Bundle By Name(cluster=w322, "Sum of Gates Graph Event Registration Refnum"=w319) -> (w321:T22)
      }
      event Mouse Leave {
        n149 = event-data() -> ("CtlRef"=w324:refnum<vi>)  [unwired: 1 in]
        n150 = Unbundle By Name(w328) -> ("f(tau) Graph Event Registration Refnum"=w326:refnum<event-registration>)
        n151 = call "XY Graph Tipstrip Mouse Leave.vi"("Event Registration Refnum"=w326, "XY Graph Refnum"=w324) -> ("Event Registration Refnum"=w325:refnum<event-registration>)  [unwired: 8 in, 1 out]
        n152 = Bundle By Name(cluster=w328, "f(tau) Graph Event Registration Refnum"=w325) -> (w327:T22)
      }
      event Mouse Leave {
        n153 = event-data() -> ("CtlRef"=w330:refnum<vi>)  [unwired: 1 in]
        n154 = Unbundle By Name(w334) -> ("a(b) Graph Event Registration Refnum"=w332:refnum<event-registration>)
        n155 = call "XY Graph Tipstrip Mouse Leave.vi"("Event Registration Refnum"=w332, "XY Graph Refnum"=w330) -> ("Event Registration Refnum"=w331:refnum<event-registration>)  [unwired: 8 in, 1 out]
        n156 = Bundle By Name(cluster=w334, "a(b) Graph Event Registration Refnum"=w331) -> (w333:T22)
      }
      event Mouse Leave {
        n157 = event-data() -> ("CtlRef"=w336:refnum<vi>)  [unwired: 1 in]
        n158 = Unbundle By Name(w340) -> ("Pseudo-Phase Lifetime Graph Event Registration Refnum"=w338:refnum<event-registration>)
        n159 = call "XY Graph Tipstrip Mouse Leave.vi"("Event Registration Refnum"=w338, "XY Graph Refnum"=w336) -> ("Event Registration Refnum"=w337:refnum<event-registration>)  [unwired: 8 in, 1 out]
        n160 = Bundle By Name(cluster=w340, "Pseudo-Phase Lifetime Graph Event Registration Refnum"=w337) -> (w339:T22)
      }
      event Mouse Leave {
        n161 = event-data() -> ("CtlRef"=w342:refnum<vi>)  [unwired: 1 in]
        n162 = Unbundle By Name(w346) -> ("Decay & Gate Graph Event Registration Refnum"=w344:refnum<event-registration>)
        n163 = call "XY Graph Tipstrip Mouse Leave.vi"("Event Registration Refnum"=w344, "XY Graph Refnum"=w342) -> ("Event Registration Refnum"=w343:refnum<event-registration>)  [unwired: 8 in, 1 out]
        n164 = Bundle By Name(cluster=w346, "Decay & Gate Graph Event Registration Refnum"=w343) -> (w345:T22)
      }
      event Mouse Move {
        n165 = event-data() -> ("CtlRef"=w349:refnum<vi>, "Coords"=w348:T26)  [unwired: 1 in]
        n166 = call "XY Graph TipStrip Mouse Move.vi"("Coords"=w348, "XY Graph Refnum"=w349) -> ()  [unwired: 7 in, 3 out]
      }
      event "Show UC Ticks": Value Change {
        n167 = event-data() -> ("NewVal"=w353:bool)  [unwired: 1 in]
        n168 = Bundle By Name(cluster=T20 {"SEPXP Q Event"=enum."Show-Hide UC Ticks", "Data"=variant} ("element"), "Data"=w353) -> (w352:T20)
        n169 = Build Array(w352) -> (w351:T20[])
        n170 = Enqueue Element(queue=w355, element=w351) -> ()  [unwired: 2 in, 3 out]
      }
      event "Phasor Graph": Cursor Move {
        n171 = event-data() -> ("CtlRef"=w358:refnum<vi>, "CursIdx"=w364:i32, "CursRef"=w359:refnum<vi>, "PlotIdx"=w363:i32, "PointIdx"=w362:i32, "CursLoc"=w361:cluster{"X":dbl, "Y":dbl})  [unwired: 1 in]
        n172 = Bundle By Name(cluster=T24 {"CtlRef"=refnum, "CursIdx"=0, "CursRef"=refnum, "PlotIdx"=0, "PointIdx"=0, "CursLoc"={"X"=0.0, "Y"=0.0}} ("output cluster"), "CtlRef"=w358, "CursIdx"=w364, "CursRef"=w359, "PlotIdx"=w363, "PointIdx"=w362, "CursLoc"=w361) -> (w360:T24)
        n173 = Bundle By Name(cluster=T20 {"SEPXP Q Event"=enum."Update Phase & Modulus Lifetime", "Data"=variant} ("element"), "Data"=w360) -> (w366:T20)
        n174 = Build Array(w366) -> (w365:T20[])
        n175 = Enqueue Element(queue=w368, element=w365) -> ()  [unwired: 2 in, 3 out]
      }
      event "Phasor Graph", "Sum of Gates Graph", "Decay & Gates Graph", "f(tau) Graph", "a(b) Graph", "Pseudo-Phase Lifetime Graph": Shortcut Menu Selection (User) {
        n176 = event-data() -> ("ItemTag"=w370:string, "CtlRef"=w375:refnum<vi>, "Coords"=w374:T26)  [unwired: 1 in]
        n177 = Bundle("ItemTag"=w370, "CtlRef"=w375, "Coords"=w374) -> (w376:T31)  [unwired: 1 in]
        n178 = call "Is XY Graph Special Event.vi"("XY Graph Event"=w376) -> ("XY Graph Event"=w372:T25, "Special Event"=w373:bool)  [unwired: 8 in, 1 out]
        n179 = case shown="False" w373 {
          tunnel: w372 -> [w377 w392]
          tunnel: w371 -> [w378 w394]
          tunnel: w370 -> [w379 _]
          frame False {
            n180 = case shown="\"Fit to Circle\"" w379 {
              tunnel: w378 -> [_ w388]
              tunnel: w377 -> [_ w389]
              frame "", Default {
              }
              frame "Fit to Circle" {
                n181 = Unbundle(w389) -> ("CtlRef"=w384:refnum<vi>, "Coords"=w383:T26)  [unwired: 1 out]
                n182 = Bundle(cluster=T28 {"XY Graph Ref"=refnum, "Mouse Coordinates"={"X"=0.0, "Y"=0.0}, "Plot Index"=0} ("data"), "XY Graph Ref"=w384, "Mouse Coordinates"=w383, "Plot Index"=-1) -> (w382:T28)
                n183 = Bundle By Name(cluster=T20 {"SEPXP Q Event"=enum."Fit to Circle", "Data"=variant} ("element"), "Data"=w382) -> (w386:T20)
                n184 = Build Array(w386) -> (w385:T20[])
                n185 = Enqueue Element(queue=w388, element=w385) -> ()  [unwired: 2 in, 3 out]
              }
            }
          }
          frame True {
            n186 = Bundle By Name(cluster=T20 {"SEPXP Q Event"=enum."XY Graph Special Event", "Data"=variant} ("element"), "Data"=w392) -> (w391:T20)
            n187 = Build Array(w391) -> (w390:T20[])
            n188 = Enqueue Element(queue=w394, element=w390) -> ()  [unwired: 2 in, 3 out]
          }
        }
      }
      event Menu Selection (User) {
        n189 = event-data() -> ("ItemTag"=w401:string)  [unwired: 1 in]
        n190 = case shown="\"Update Phasor Graph\"" w401 {
          tunnel: [T20[] [] ("element") T20[] [{"SEPXP Q Event"=enum."Edit User-defined Gate", "Data"=variant}] ("element") T20[] [{"SEPXP Q Event"=enum."Update Phasor Graph", "Data"=variant}] ("element") T20[] [{"SEPXP Q Event"=enum."Update Sum of Gates Graph", "Data"=variant}] ("element") T20[] [{"SEPXP Q Event"=enum."Compute Decay &/or Gates", "Data"=variant}] ("element") T20[] [{"SEPXP Q Event"=enum."Find Pseudo UC Intersections", "Data"=variant}] ("element") T20[] [{"SEPXP Q Event"=enum."Compute alpha(beta) Plot", "Data"=variant}] ("element") T20[] [{"SEPXP Q Event"=enum."Compute Pseudo-Phase Lifetime Plot", "Data"=variant}] ("element") T20[] [{"SEPXP Q Event"=enum."Update Graph Plots Info", "Data"=variant}] ("element") T20[] [{"SEPXP Q Event"=enum."Quit", "Data"=variant}] ("element") _ _ _] -> w399
          tunnel: [_ _ _ _ _ _ _ _ _ TRUE ("Discard?") _ _ _] -> w398
          tunnel: w397 -> [_ _ _ _ _ _ _ _ _ _ w427 _ _]
          tunnel: [w402 w404 w406 w408 w410 w412 w414 w416 w418 w420 w424 w431 w437] -> w396
          tunnel: w395 -> [w402 w404 w406 w408 w410 w412 w414 w416 w418 w420 w424 w432 w436]
          frame "", Default {
          }
          frame "Edit User-defined Gate" {
          }
          frame "Update Phasor Graph" {
          }
          frame "Update Sum of Gates Graph" {
            # "deprecated"
          }
          frame "Compute Decay &/or Gates" {
          }
          frame "Find Pseudo UC Intersections" {
            # "deprecated"
          }
          frame "Compute alpha(beta) Plot" {
            # "deprecated"
          }
          frame "Compute Pseudo-Phase Lifetime Plot" {
          }
          frame "Update Graph Plots Info" {
          }
          frame "Quit" {
          }
          frame "Notebook" {
            n191 = global write "Notebook Main VI Name.vi" "Main VI Name"(w427) -> ()
            n192 = vi-ref "Notebook.vi"() -> (w429:refnum<vi>)
            n193 = property class="VI"(reference=w429) -> (error out=w428:errorcluster, "Path"=w423:path)  [unwired: 1 in, 1 out]
            n194 = Empty String/Path?(string/path=w427) -> (empty?=w426:bool)
            n195 = Not(x=w426) -> (.not. x?=w425:bool)
            n196 = call "Run Vi.vi"("VI Path"=w423, "error in (no error)"=w428, "Start Hidden? (F)"=w425) -> ()  [unwired: 5 in, 2 out]
          }
          frame "Settings" {
            n197 = vi-ref "Phasor Explorer Settings Window.vi"() -> (w434:refnum<vi>)
            n198 = property class="VI"(reference=w434) -> (error out=w433:errorcluster, "Path"=w430:path)  [unwired: 1 in, 1 out]
            n199 = call "Run Vi.vi"("VI Path"=w430, "error in (no error)"=w433) -> ()  [unwired: 6 in, 2 out]
            n200 = call "8a583f86-e298-41fd-bd3d-00e17bb4994f.vi"("Element"=w430, "Array in"=w432) -> ("Array out"=w431:path[])  [unwired: 9 in]
          }
          frame "About" {
            n201 = vi-ref "About Phasor Explorer.vi"() -> (w439:refnum<vi>)
            n202 = property class="VI"(reference=w439) -> (error out=w438:errorcluster, "Path"=w435:path)  [unwired: 1 in, 1 out]
            n203 = call "Run Vi.vi"("VI Path"=w435, "error in (no error)"=w438, "Start Hidden? (F)"=TRUE) -> ()  [unwired: 5 in, 2 out]
            n204 = call "1c9cba52-9257-43c1-b566-a5a99626e4a7.vi"("Element"=w435, "Array in"=w436) -> ("Array out"=w437:path[])  [unwired: 9 in]
          }
        }
        n205 = Enqueue Element(queue=w400, element=w399) -> ()  [unwired: 2 in, 3 out]
      }
    }
  }
  n206 = control-ref of="Display Tabs"() -> (w5:refnum<vi>)
  n207 = property class="TabCtl (strict)"(reference=w5) -> ("Pages"=w4:refnum<vi>[])  [unwired: 1 in, 2 out]
  n208 = for {
    tunnel: w4 -> [w442] mode=indexing
    tunnel: bool[] [TRUE, FALSE, FALSE, TRUE, TRUE, FALSE, FALSE] ("Page Visible") -> [w441] mode=indexing
    n209 = property class="Page"(reference=w442, "PageVis"=w441) -> ()  [unwired: 1 in, 2 out]
  }
  n210 = case shown="\"Phasor Plot\", Default" "Display Tabs" {
    frame "Phasor Plot", Default {
    }
    frame "Sum of Gates" {
    }
    frame "UC Intersections" {
    }
    frame "Alpha vs Beta" {
    }
    frame "Pseudo Phase Lifetime" {
    }
    frame "Decay, Gate & Gated Decay" {
    }
  }
  n211 = Release Queue(queue=w33) -> (error out=w27:errorcluster)  [unwired: 2 in, 2 out]
  n212 = case shown="True" w2 {
    tunnel: w27 -> [_ w448]
    tunnel: w6 -> [_ w450]
    tunnel: w1 -> [_ w449]
    frame False {
    }
    frame True {
      n213 = property class="VI"(reference=w449, error in=w448) -> (reference out=w445:refnum<vi>, error out=w444:errorcluster, "Path"=w446:path)
      n214 = Build Array (concatenate)(w450, w446) -> (w447:path[])
      n215 = Close Reference(reference=w445, error in (no error)=w444) -> (error out=w443:errorcluster)
      n216 = call "Close & Abort VIs.vi"("Error In"=w443, "VI Paths"=w447) -> ()  [unwired: 9 in, 1 out]
    }
  }
